vi "Fetch Rx Data (I16).vi"(0 "Register Bus":T1, 2 "vertical range [Vpp]":dbl=2.0 format="%#_6p", 5 "number of samples":u32=8196, 9 "timeout [s]":dbl=10.0, 11 "error in":errorcluster, 13 "leading samples to trim":i32) -> (3 "scaling (V/code)":dbl, 4 "Register Bus (out)":T1, 6 "waveform data":i16[](array[numeric]), 15 "error out":errorcluster)   [LabVIEW 2017]
doc: "Fetch Rx data from the device. It's required to call <b>Configure Stream</b> and <b>Initiate Stream</b> before calling this VI."
uses:
  <instrlib>/_niInstr/Register Bus/v0/Host/Public/Register Bus Session.ctl
  <instrlib>/_niInstr/Register Bus/v0/Host/Private/Session Data.ctl
  Rx FPGA VI Reference.ctl
  <vilib>/rvi/errors/niLvFpgaAdjustHostInterfaceError.vi
  <vilib>/rvi/interface/nirviMethod/nirviMethod.xnode
  <instrlib>/_niInstr/Register Bus/v0/Host/niInstr Register Bus v0 Host.lvlib
  <vilib>/FPGAPlugInAG/Dynamic/niLvFpga_ReadFifo_Dynamic.vi
  <vilib>/rvi/errors/niLvFpgaMergeErrorWithErrorCode.vi
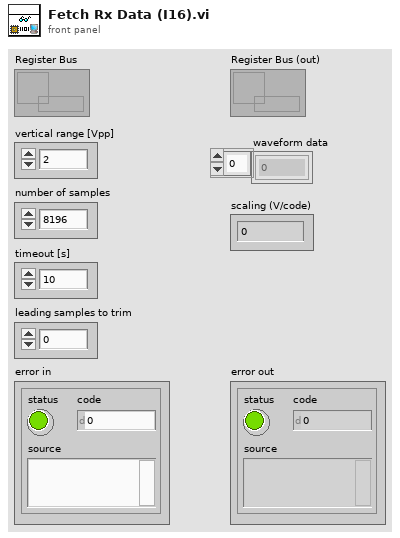
[diagram p1: front panel]
types:
  T1 = typedef "niInstr Register Bus v0 Host.lvlib/Register Bus Session.ctl" = refnum<queue>
  T2 = typedef "Rx FPGA VI Reference.ctl" = refnum<k20>
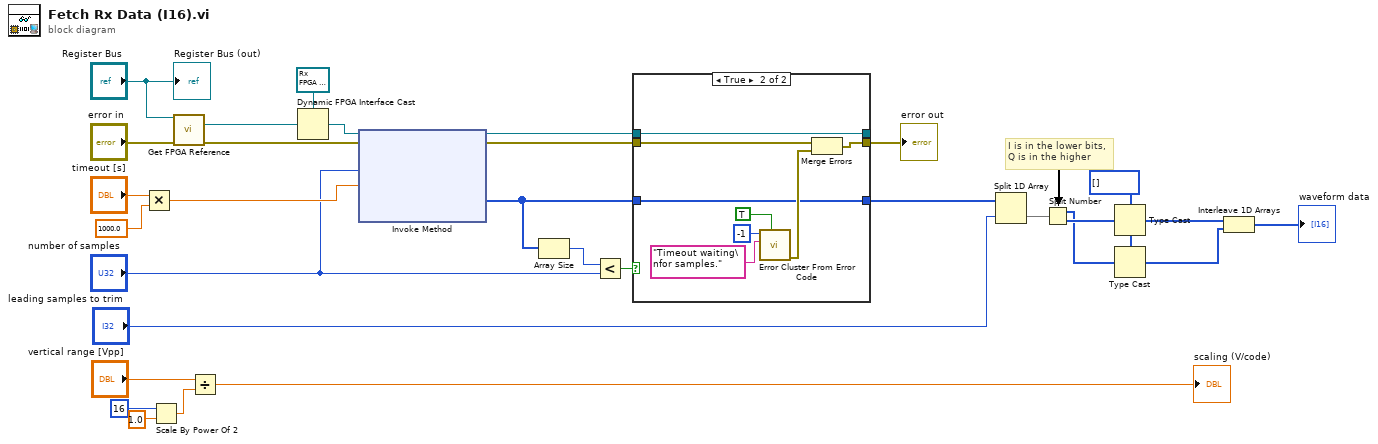
[diagram p0: block diagram]
diagram:
  w10 = i16[] []
  # "I is in the lower bits,\nQ is in the higher"
  n1 = Multiply(x="timeout [s]", y=1000.0) -> (x*y=w21:dbl)
  n2 = Scale By Power Of 2(n=i16 16 ("ADC Resolution (bits)"), x=1.0) -> (x*2^n=w13:dbl)
  n3 = call <instrlib>:"Get FPGA Reference.vi"("session in"="Register Bus", "error in"="error in") -> ("fpga ref"=w28:refnum<k20>, "error out"=w27:errorcluster)  [unwired: 11 in, 1 out]
  n4 = Divide(x="vertical range [Vpp]", y=w13) -> (x/y=→"scaling (V/code)":dbl)
  n5 = Dynamic FPGA Interface Cast(Session In=T2 refnum ("Type"), Type=w28) -> (Session Out=w26:T2)
  n6 = xnode "Invoke Method"("FPGA VI Reference In"=w26, "error in"=w27, "Number of Elements"="number of samples", "Timeout (ms)"=w21) -> ("FPGA VI Reference Out"=w24:T2, "error out"=w25:errorcluster, "Data"=w6:u32[])  [unwired: 1 out]
  n7 = Array Size(array=w6) -> (size(s)=w5:i32)
  n8 = Less?(x=w5, y="number of samples") -> (x < y?=w19:bool)
  n9 = case shown="True" w19 {
    tunnel: w24 -> [w33 w41]
    tunnel: w25 -> [w32 w38]
    tunnel: [w33 w41] -> _
    tunnel: [w32 w37] -> w17
    tunnel: [w31 w34] -> w4
    tunnel: w6 -> [w31 w34]
    frame False {
    }
    frame True {
      n10 = call <vilib>:"Error Cluster From Error Code.vi"("show call chain? (False)"=TRUE, "error message (\"\")"="Timeout waiting\nfor samples." ("error message (\"\")"), "error code (0)"=-1) -> ("error out"=w36:errorcluster)  [unwired: 6 in]
      n11 = Merge Errors(w38, w36) -> (w37:errorcluster)
    }
  }
  "error out" <- w17
  n12 = Split 1D Array(array=w4, index="leading samples to trim") -> (second subarray=w9:u32[])  [unwired: 1 out]
  n13 = Split Number(x=w9) -> (hi(x)=w7:u16[], lo(x)=w8:u16[])
  n14 = Type Cast(type=w10, x=w8) -> (*(type *) &x=w3:i16[])
  n15 = Type Cast(type=w10, x=w7) -> (*(type *) &x=w2:i16[])
  n16 = Interleave 1D Arrays(w3, w2) -> (→"waveform data":i16[])
  "Register Bus (out)" <- "Register Bus"
